vi "CheckValidProgram.vi"(8 "loadedProgram in":string) -> (0 "loadedProgram out":string, 2 "valid?":bool)   [LabVIEW 2016, in "Universal Robot.lvclass"]
uses:
  Universal Robot.lvclass
  <vilib>/regexp/Match Regular Expression.xnode
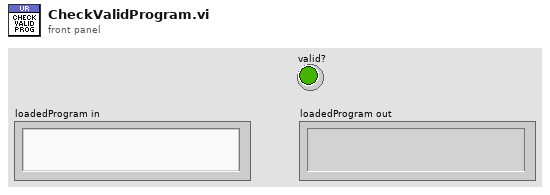
[diagram p1: front panel]
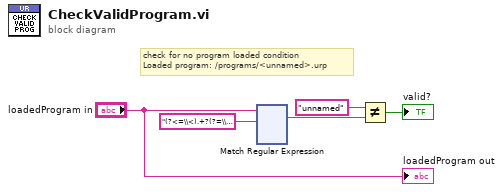
[diagram p0: block diagram]
diagram:
  # "check for no program loaded condition\nLoaded program: /programs/<unnamed>.urp"
  n1 = xnode "Match Regular Expression"("input string"="loadedProgram in", "regular expression"="(?<=\\<).+?(?=\\>)") -> ("whole match"=w1:string)  [unwired: 4 in, 4 out]
  n2 = Not Equal?(x="unnamed", y=w1) -> (x != y?=→"valid?":bool)
  "loadedProgram out" <- "loadedProgram in"
